vi "URLRoot.vi"(11 "URL":string) -> (2 "Root Name":string, 3 "URL Dup":string)   [LabVIEW 2017, in "TagDB.lvlib"]
uses:
  TagDB.lvlib
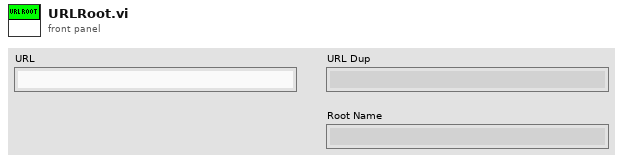
[diagram p1: front panel]
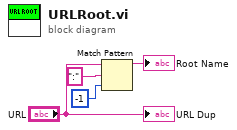
[diagram p0: block diagram]
diagram:
  n1 = Match Pattern(string="URL", regular expression=":", offset (0)=-1) -> (before substring=→"Root Name":string)  [unwired: 3 out]
  "URL Dup" <- "URL"
